vi "4~20mA 10bar.vi"(1 "Current mA":dbl) -> (0 "Pressure bar":dbl)   [LabVIEW 2024]
doc: "Scale the 4-20mA to 0-10 bar range."
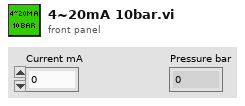
[diagram p1: front panel]
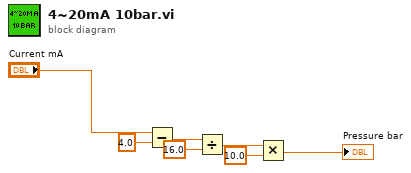
[diagram p0: block diagram]
diagram:
  n1 = Subtract(x="Current mA", y=4.0) -> (x-y=w3:dbl)
  n2 = Divide(x=w3, y=16.0) -> (x/y=w5:dbl)
  n3 = Multiply(x=w5, y=10.0) -> (x*y=→"Pressure bar":dbl)
